vi "PDE_Evaluate Steady 2D Func.vi"(7 "data":variant, 8 "error in (no error)":errorcluster, 9 "Y":dbl[](array[numeric]), 10 "X":dbl[](array[numeric]), 11 "VIRef":refnum<vi>) -> (0 "error out":errorcluster, 3 "F(x, y)":dbl[][](array[numeric]))   [LabVIEW 2017, in "NI_PDE.lvlib"]
uses:
  <vilib>/gmath/NI_PDE.lvlib
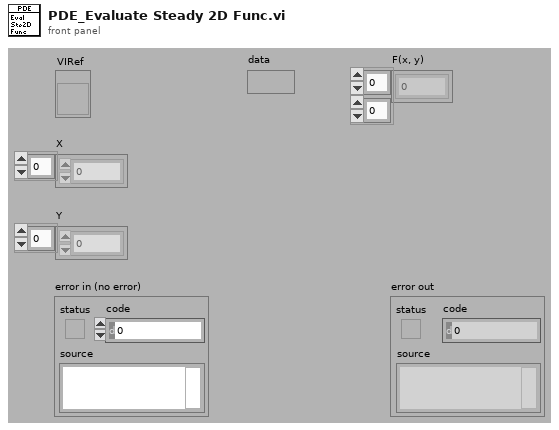
[diagram p1: front panel]
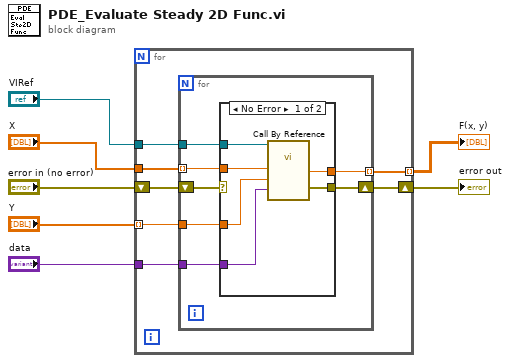
[diagram p0: block diagram]
diagram:
  n1 = for {
    tunnel: "X" -> [w12]
    tunnel: "Y" -> [w14] mode=indexing
    tunnel: "VIRef" -> [w13]
    tunnel: "data" -> [w11]
    shift-right: [w10] -> w5
    shift-left: "error in (no error)" -> [w9]
    tunnel: [w8] -> w3 mode=indexing
    n2 = for {
      tunnel: w14 -> [w19]
      tunnel: w13 -> [w21]
      tunnel: w12 -> [w20] mode=indexing
      tunnel: w11 -> [w18]
      shift-right: [w17] -> w10
      shift-left: w9 -> [w16]
      tunnel: [w15] -> w8 mode=indexing
      n3 = case shown="No Error" w16 {
        selector: w16 -> [_ w28]
        tunnel: w21 -> [w27 _]
        tunnel: w20 -> [w26 _]
        tunnel: w19 -> [w25 _]
        tunnel: w18 -> [w24 _]
        tunnel: [w23 w28] -> w17
        tunnel: [w22 _] -> w15
        frame No Error {
          n4 = call-by-ref "?"(reference=w27, "data"=w24, "y"=w25, "x"=w26) -> ("error out"=w23:errorcluster, "f(x, y)"=w22:dbl)  [unwired: 1 in, 2 out]
        }
        frame Error {
        }
      }
    }
  }
  "F(x, y)" <- w3
  "error out" <- w5
